vi "Apply General Configuration.vi"(7 "Restart (T)":bool=TRUE, 8 "error in (no error)":errorcluster, 10 "Protocol (Legacy)":T1, 11 "Ethernet in":refnum<class "ENET_BS120x.lvclass">) -> (0 "error out":errorcluster, 3 "Ethernet out":refnum<class "ENET_BS120x.lvclass">)   [LabVIEW 2021, in "BS120x Driver.lvlib" / "ENET_BS120x.lvclass"]
doc: "DEPRECATED for BS1201 \nno general config anymore; BS1201 can handle ENET and CAN at the same time.\nENET has ability to disable broadcast"
uses:
  ENET_BS120x.lvclass
  TypeDefs/Protocol.ctl
  BS120x.lvclass
panel:
  # "no general config anymore; BS1201 can handle ENET and CAN at the same time.\nENET has ability to disable broadcast"
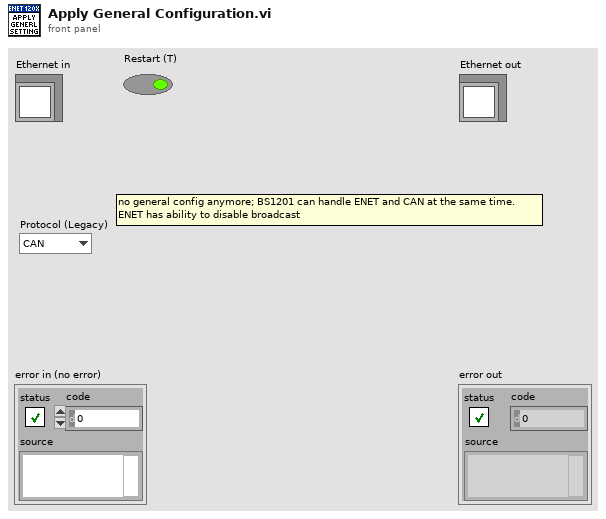
[diagram p1: front panel]
types:
  T1 = typedef "BS120x Driver.lvlib/BS120x.lvclass/Protocol.ctl" = enum16{"CAN", "Ethernet"}
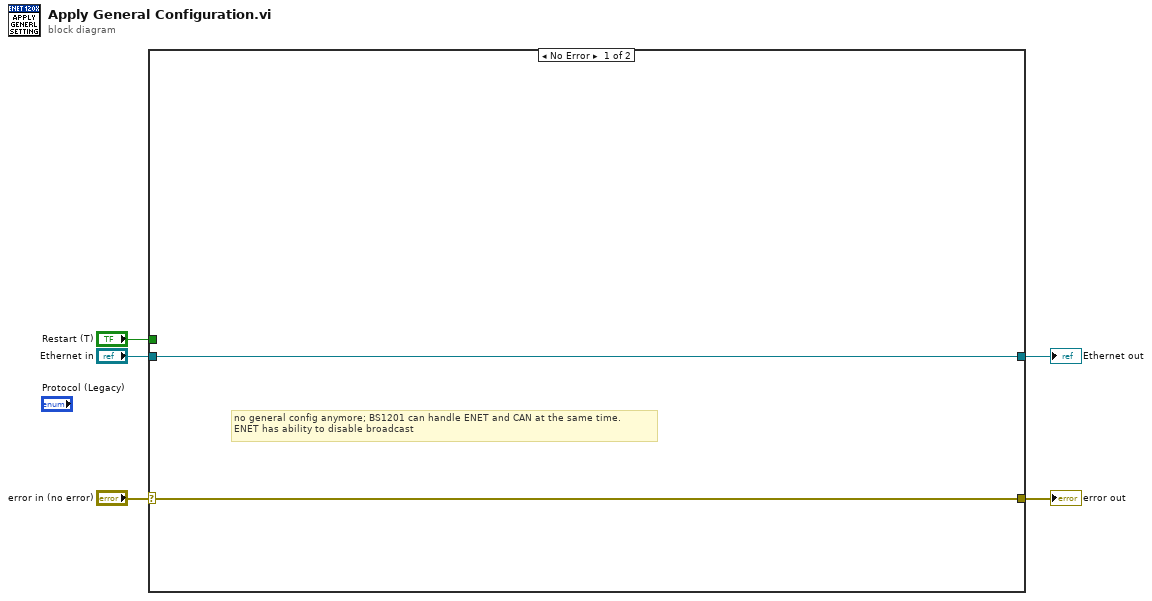
[diagram p0: block diagram]
diagram:
  n1 = case shown="No Error" "error in (no error)" {
    selector: "error in (no error)" -> [w6 w9]
    tunnel: [w6 w9] -> w4
    tunnel: [w7 w8] -> w2
    tunnel: "Ethernet in" -> [w7 w8]
    tunnel: "Restart (T)" -> [_ _]
    frame No Error {
      # "no general config anymore; BS1201 can handle ENET and CAN at the same time.\nENET has ability to disable broadcast"
    }
    frame Error {
    }
  }
  "error out" <- w4
  "Ethernet out" <- w2
